vi "Update UI State.vi"(11 "Busy":bool) -> (2 "Disabled 2":T1(ring), 3 "Disabled":T1(ring))   [LabVIEW 2022 SP3, in "DAQ View.lvclass"]
uses:
  DAQ View.lvclass
  DAQ View.lvclass/DAQ View.ctl
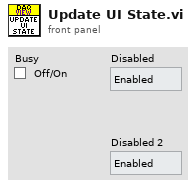
[diagram p1: front panel]
types:
  T1 = enum8{"Enabled", "Disabled", "Disabled and Grayed Out"}
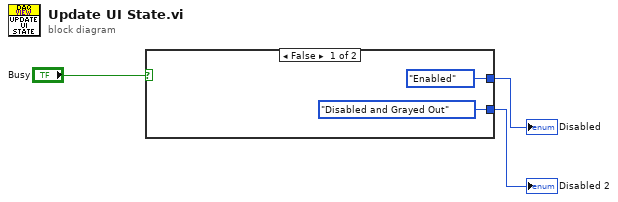
[diagram p0: block diagram]
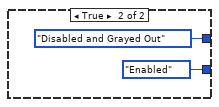
[diagram p2: hidden frame]
diagram:
  n1 = case shown="False" "Busy" {
    tunnel: [T1."Disabled and Grayed Out" ("Disabled") T1."Enabled" ("Disabled")] -> w2
    tunnel: [T1."Enabled" ("Disabled") T1."Disabled and Grayed Out" ("Disabled")] -> w3
    frame False {
    }
    frame True {
    }
  }
  "Disabled" <- w3
  "Disabled 2" <- w2
